vi "Unlock Drive.vi"(8 "error in":errorcluster, 10 "Force":bool, 11 "Queue in":refnum<queue>) -> (0 "error out":errorcluster)   [LabVIEW 2016, in "Drive System.lvlib"]
uses:
  Drive System.lvlib
  DriveCmd.ctl
  DriveCmdList.ctl
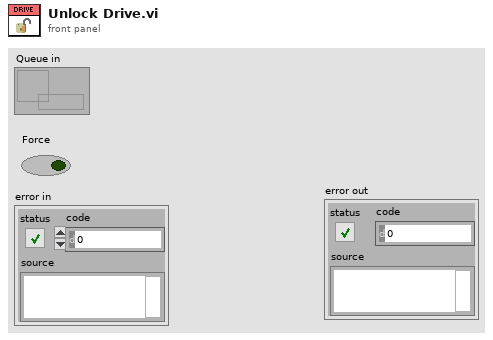
[diagram p1: front panel]
types:
  T1 = typedef "Drive System.lvlib/DriveCmd.ctl" = cluster{"cmd":T2, "data":variant, "Force? (F)":bool, "Lock":string}
  T2 = typedef "Drive System.lvlib/DriveCmdList.ctl" = enum16{"Idle", "Cleanup", "Drive For Time", "Drive Tank", "Drive Arcade", "Unlock", "Lock"}
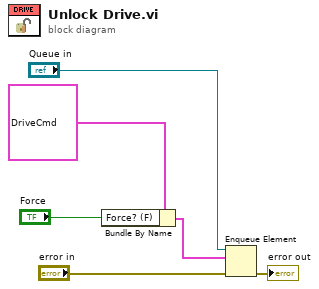
[diagram p0: block diagram]
diagram:
  n1 = Bundle By Name(cluster=T1 {"cmd"=enum."Unlock", "data"=variant, "Force? (F)"=FALSE, "Lock"=""} ("element"), "Force? (F)"="Force") -> (w1:T1)
  n2 = Enqueue Element(queue="Queue in", element=w1, error in (no error)="error in") -> (error out=→"error out":errorcluster)  [unwired: 1 in, 2 out]
